vi "DiscreteHys.vi"(1 "DBO Para":T1, 2 "En H":bool, 3 "input x":dbl[](array[numeric])=[0.0, 0.0, 0.0]) -> (0 "Y":dbl[](array[numeric]))   [LabVIEW 2011]
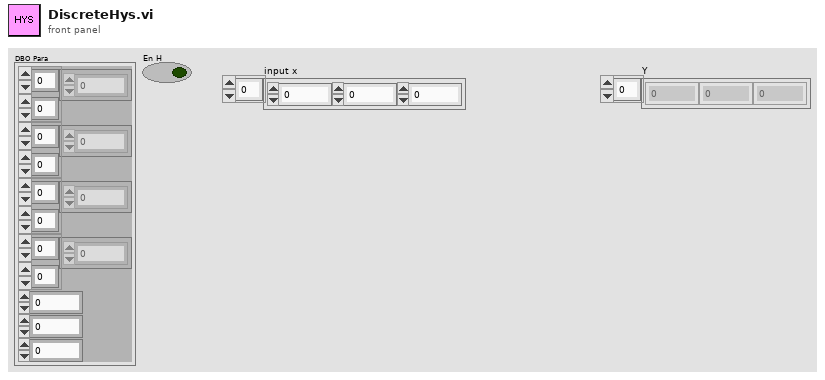
[diagram p1: front panel]
types:
  T1 = cluster{dbl[][], dbl[][], dbl[][], dbl[][], dbl, dbl, dbl}
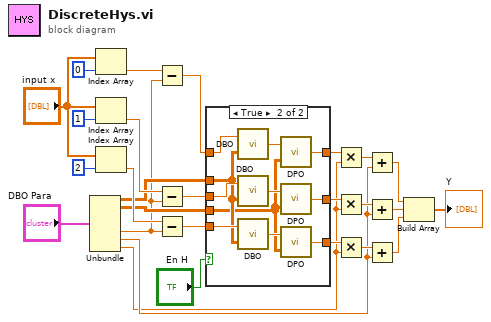
[diagram p0: block diagram]
diagram:
  n1 = Unbundle("DBO Para") -> (w6:dbl[][], w5:dbl[][], w4:dbl, w3:dbl, w2:dbl)  [unwired: 2 out]
  n2 = Index Array(array="input x", index=0) -> (element=w20:dbl)
  n3 = Index Array(array="input x", index=1) -> (element=w18:dbl)
  n4 = Index Array(array="input x", index=2) -> (element=w16:dbl)
  n5 = Subtract(x=w20, y=w4) -> (x-y=w19:dbl)
  n6 = Subtract(x=w18, y=w4) -> (x-y=w17:dbl)
  n7 = Subtract(x=w16, y=w4) -> (x-y=w15:dbl)
  n8 = case shown="True" "En H" {
    tunnel: w19 -> [w30 w40]
    tunnel: w17 -> [w29 w39]
    tunnel: w15 -> [w28 w38]
    tunnel: [w30 w35] -> w10
    tunnel: [w29 w34] -> w9
    tunnel: [w28 w33] -> w8
    tunnel: w6 -> [_ w32]
    tunnel: w5 -> [_ w31]
    frame False {
    }
    frame True {
      n9 = call "DBO.vi"("H"=w32, "x"=w40) -> ("y"=w41:dbl)
      n10 = call "DBO.vi"("H"=w32, "x"=w39) -> ("y"=w36:dbl)
      n11 = call "DBO.vi"("H"=w32, "x"=w38) -> ("y"=w37:dbl)
      n12 = call "DPO.vi"("S"=w31, "x"=w41) -> ("y"=w35:dbl)
      n13 = call "DPO.vi"("S"=w31, "x"=w36) -> ("y"=w34:dbl)
      n14 = call "DPO.vi"("S"=w31, "x"=w37) -> ("y"=w33:dbl)
    }
  }
  n15 = Multiply(x=w10, y=w2) -> (x*y=w22:dbl)
  n16 = Multiply(x=w9, y=w2) -> (x*y=w12:dbl)
  n17 = Multiply(x=w8, y=w2) -> (x*y=w14:dbl)
  n18 = Add(x=w22, y=w3) -> (x+y=w21:dbl)
  n19 = Add(x=w12, y=w3) -> (x+y=w11:dbl)
  n20 = Add(x=w14, y=w3) -> (x+y=w13:dbl)
  n21 = Build Array(w21, w11, w13) -> (→"Y":dbl[])
